vi "Host - Laptop.vi"() -> ()   [LabVIEW 2017]
uses:
  sobot structures/Commands.ctl
  sobot structures/General_Command.ctl
  sobot structures/ReturnDataStatus.ctl
  sobot structures/XY_Commands.ctl
  sobot structures/Z_Command.ctl
  1dab9ac5-030c-4d51-9c07-0e0460f9bdda.vi
  45e61c1e-af3e-4776-95f2-28021f87d7f5.vi
  209d0eb8-92f5-4172-9cd1-3ed4126d6dd2.vi
  fabacc7d-1012-48c4-9930-a2795e4d71c6.vi
  f1c2f41c-6d0d-4fd5-9c33-fd296998c35a.vi
  567dd2d4-847b-4f17-917f-034123e5cef3.vi
  5a9a0e87-71f9-401a-87e2-2bb0dd87a38c.vi
  200908e3-6be4-4c90-a5fc-498c46c2d1bf.vi
  6d8adddc-4429-438c-b8f0-ba7b589ea023.vi
  c3afd2a6-b29d-4eb4-b88f-7abd21b0c47a.vi
  5fae1378-0665-4254-b68d-0e395951aabf.vi
  267ce563-aefe-4b16-b1f3-47eae334334f.vi
  99eac005-18d9-4fd3-997a-104f87d8fe48.vi
  20e12de9-b1e8-45fd-8220-b65a0c4cd02e.vi
  82c37991-5cff-4107-993c-edab275d39a1.vi
  27a68409-aeb0-4d2d-83e9-8f13cebcd619.vi
  de5fd1d6-9d33-402c-82a6-f57f77f69c7e.vi
  29953faf-593d-4707-840b-6a073ddb8916.vi
panel:
  out "Pingtime":i32
  in  "General_Ping":bool
  out "String":string
  in  "ReflectorPosition":i32
  in  "Z_Position":i32
  in  "Z_Focus":bool
  in  "Z_Initialize":bool
  in  "Z_ReflectorPosition":bool
  in  "Z_MoveToPosition":bool
  in  "XY_Unlock Motors":bool
  in  "XY_LockMotors":bool
  in  "XY_MarkTarget":bool
  in  "XY_MoveToPosition":bool
  in  "XY_Initialize":bool
  in  "Coordinate":dbl[](array[numeric])=[0.0, 0.0, 0.0]
  in  "Message":string
  in  "Positon (X / Y)":i32[](array[numeric])
  in  "General_SimpleMessage":bool
  in  "General_Initialize":bool
  in  "General_TransferPoint":bool
  in  "General_StopSobotAutomatic":bool
  in  "General_StartSobotAutomatic":bool
  in  "General_Stop":bool
  # "General"
  # "XY"
  # "Z"
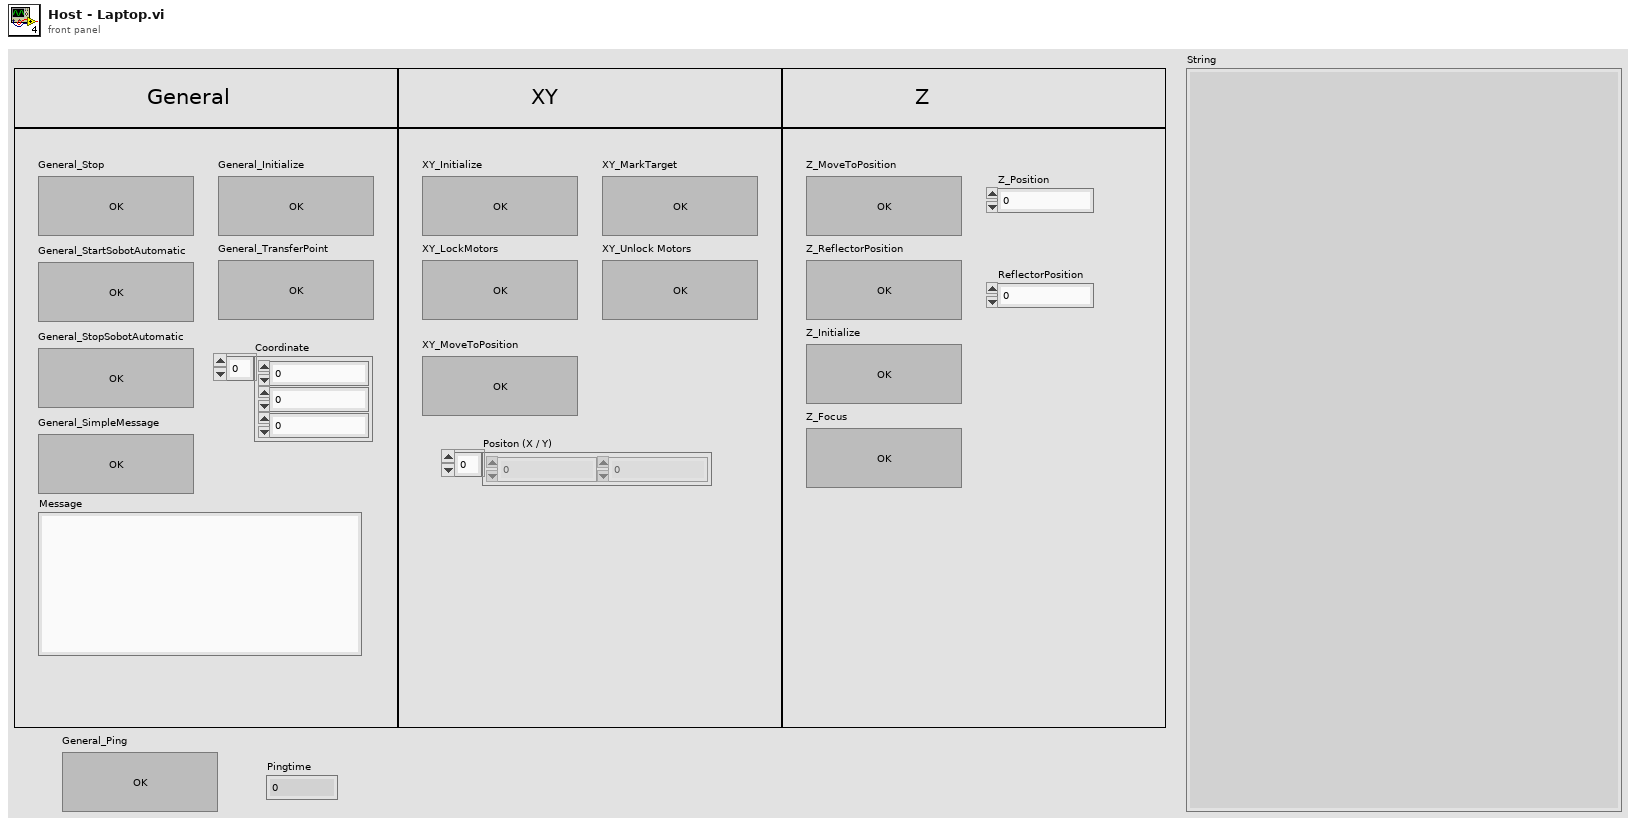
[diagram p1: front panel]
types:
  T1 = typedef "Commands.ctl" = enum16{"General_Stop", "General_StartSobotAutomatic", "General_StopSobotAutomatic", "General_TransferPoint", "General_Initialize", "General_SimpleMessage", "General_Ping", "XY_Initialize", "XY_MoveToPosition", "XY_MarkTarget", "XY_LockMotors", "XY_UnlockMotors", "Z_Initialize", "Z_MoveToPosition", "Z_Focus", "Z_ReflectorPosition", "Plattform_Move", "Plattform_GetDrivingData", "Plattform_GetLivetimeData"}
  T2 = typedef "General_Command.ctl" = enum16{"General_Stop", "General_StartSobotAutomatic", "General_StopSobotAutomatic", "General_TransferPoint", "General_Initialize", "General_SimpleMessage", "General_Ping"}
  T3 = typedef "ReturnDataStatus.ctl" = enum16{"AllOk", "Error"}
  T4 = typedef "XY_Commands.ctl" = enum16{"XY_Initialize", "XY_MoveToPosition", "XY_MarkTarget", "XY_LockMotors", "XY_UnlockMotors"}
  T5 = typedef "Z_Command.ctl" = enum16{"Z_Initialize", "Z_MoveToPosition", "Z_Focus", "Z_ReflectorPosition"}
  T6 = typedef "SoBot_CommandTypes.ctl" = enum16{"General_Command", "XY_Command", "Z_Command", "Plattform_Command"}
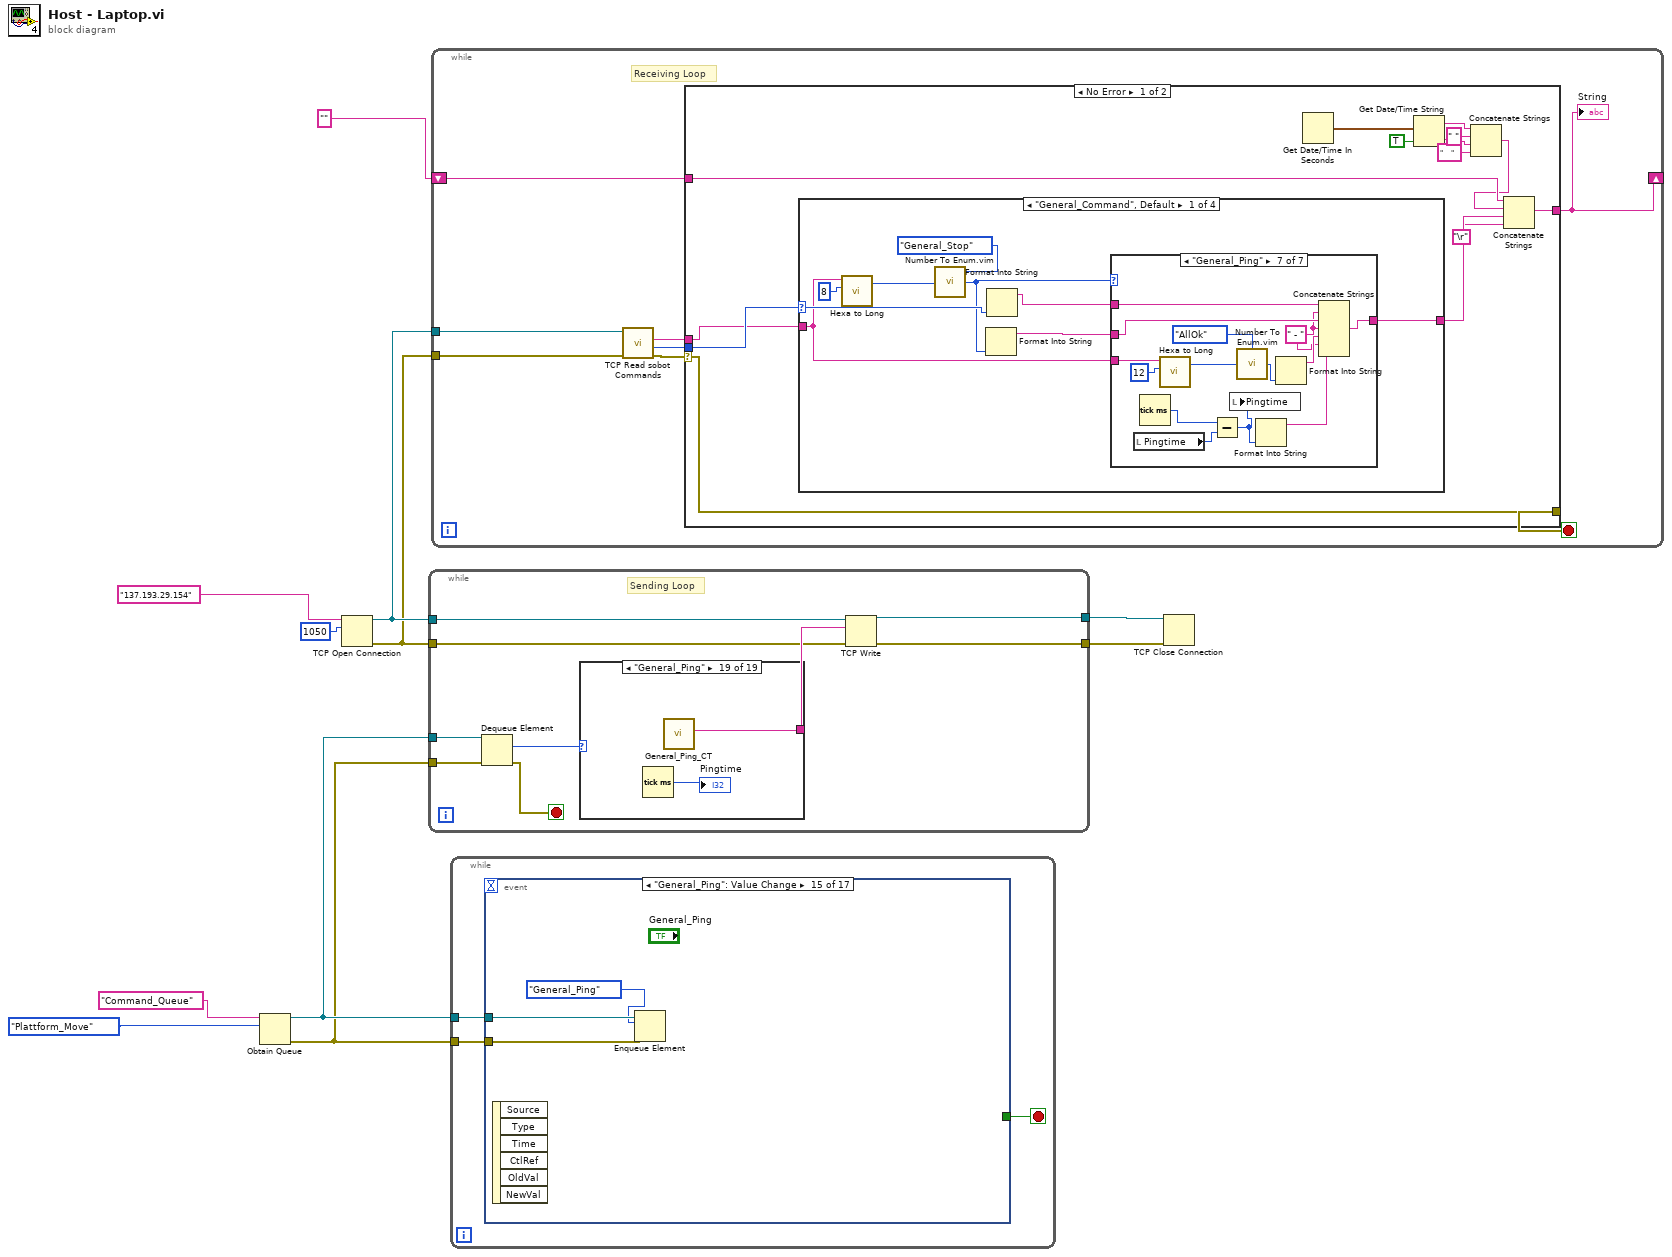
[diagram p0: block diagram]
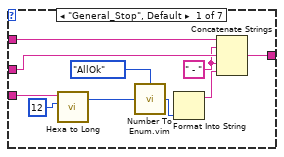
[diagram p2: hidden frame]
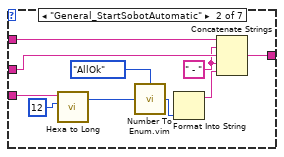
[diagram p3: hidden frame]
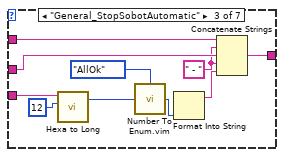
[diagram p4: hidden frame]
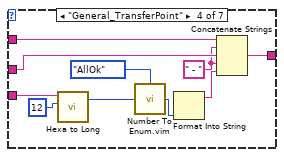
[diagram p5: hidden frame]
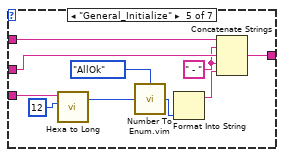
[diagram p6: hidden frame]
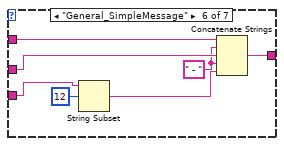
[diagram p7: hidden frame]
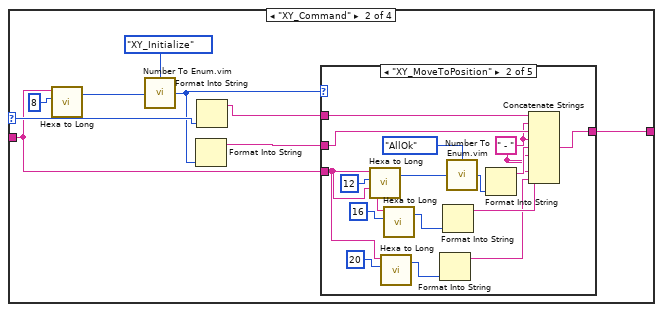
[diagram p8: hidden frame]
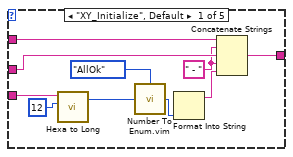
[diagram p9: hidden frame]
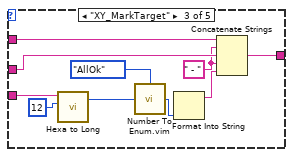
[diagram p10: hidden frame]
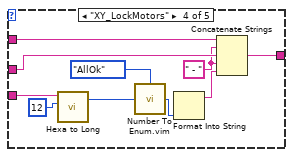
[diagram p11: hidden frame]
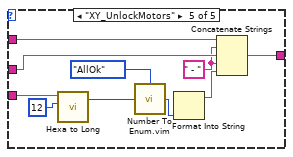
[diagram p12: hidden frame]
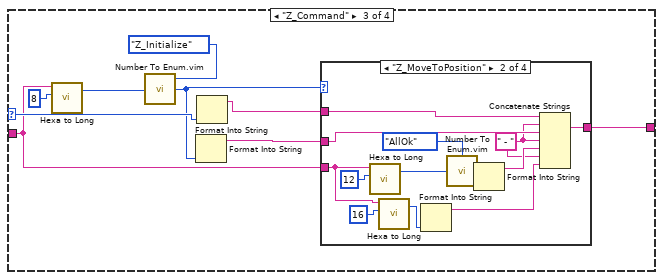
[diagram p13: hidden frame]
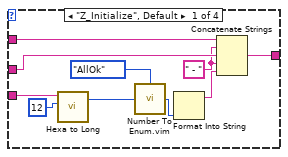
[diagram p14: hidden frame]
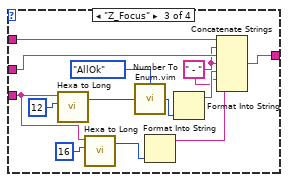
[diagram p15: hidden frame]
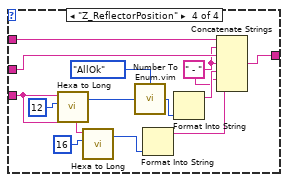
[diagram p16: hidden frame]
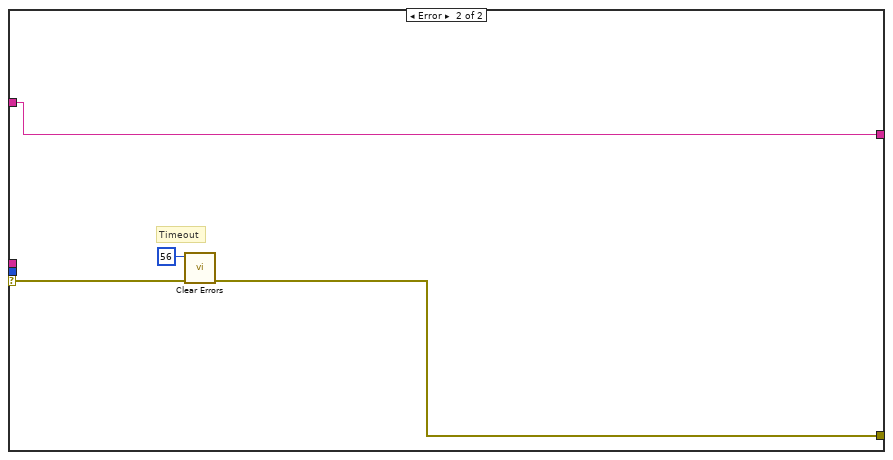
[diagram p18: hidden frame]
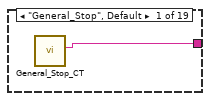
[diagram p19: hidden frame]
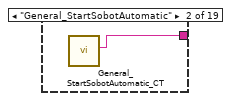
[diagram p20: hidden frame]
diagram:
  n1 = Obtain Queue(name (unnamed)="Command_Queue", element data type=Commands."Plattform_Move") -> (queue out=w7:refnum<queue>, error out=w6:errorcluster)  [unwired: 3 in, 1 out]
  n2 = TCP Open Connection(address="137.193.29.154", remote port or service name=u16 1050) -> (connection ID=w3:refnum<k5>, error out=w2:errorcluster)  [unwired: 3 in]
  n3 = while {
    tunnel: w3 -> [w15]
    tunnel: w2 -> [w14]
    tunnel: w7 -> [w19]
    tunnel: w6 -> [w20]
    tunnel: [w13] -> w5
    tunnel: [w12] -> w4
    stop <- w17 stop-if-true
    # "Sending Loop"
    n4 = Dequeue Element(queue=w19, error in (no error)=w20) -> (element=w18:T1, error out=w17:errorcluster)  [unwired: 1 in, 2 out]
    n5 = case shown="\"General_Ping\"" w18 {
      tunnel: [w21 w22 w23 w25 w26 w28 w29 w31 w32 w33 w34 w35 w37 w38 w40 w41 w42 w43 w45] -> w16
      frame "General_Stop", Default {
        n6 = call "General_Stop_CT.vi"() -> ("Command"=w21:string)  [unwired: 11 in]
      }
      frame "General_StartSobotAutomatic" {
        n7 = call "General_StartSobotAutomatic_CT.vi"() -> ("Command"=w22:string)  [unwired: 11 in]
      }
      frame "General_StopSobotAutomatic" {
        n8 = call "General_StopSobotAutomatic_CT.vi"() -> ("Command"=w23:string)  [unwired: 11 in]
      }
      frame "General_TransferPoint" {
        n9 = call "General_TransferPoint_CT.vi"("Coordinate"="Coordinate") -> ("Command"=w25:string)  [unwired: 10 in]
      }
      frame "General_Initialize" {
        n10 = call "General_Initialize_CT.vi"() -> ("Command"=w26:string)  [unwired: 11 in]
      }
      frame "General_SimpleMessage" {
        n11 = call "General_SimpleMessage_CT.vi"("Message"="Message") -> ("Command"=w28:string)  [unwired: 10 in]
      }
      frame "XY_Initialize" {
        n12 = call "XY_Initialize_CT.vi"() -> ("Command"=w29:string)  [unwired: 11 in]
      }
      frame "XY_MoveToPosition" {
        n13 = call "XY_MoveToPosition_CT.vi"("Positon (X / Y)"="Positon (X / Y)") -> ("Command"=w31:string)  [unwired: 10 in]
      }
      frame "XY_MarkTarget" {
        n14 = call "XY_MarkTarget_CT.vi"() -> ("Command"=w32:string)  [unwired: 11 in]
      }
      frame "XY_LockMotors" {
        n15 = call "XY_LockMotors_CT.vi"() -> ("Command"=w33:string)  [unwired: 11 in]
      }
      frame "XY_UnlockMotors" {
        n16 = call "XY_UnlockMotors_CT.vi"() -> ("Command"=w34:string)  [unwired: 11 in]
      }
      frame "Z_Initialize" {
        n17 = call "Z_Initialize_CT.vi"() -> ("Command"=w35:string)  [unwired: 11 in]
      }
      frame "Z_MoveToPosition" {
        n18 = call "Z_MoveToPosition_CT.vi"("Z_Position"="Z_Position") -> ("Command"=w37:string)  [unwired: 10 in]
      }
      frame "Z_Focus" {
        n19 = call "Z_Focus_CT.vi"() -> ("Command"=w38:string)  [unwired: 11 in]
      }
      frame "Z_ReflectorPosition" {
        n20 = call "Z_ReflectorPosition_CT.vi"("ReflectorPosition"="ReflectorPosition") -> ("Command"=w40:string)  [unwired: 10 in]
      }
      frame "Plattform_Move" {
        n21 = call "Plattform_Move_CT.vi"() -> ("Command"=w41:string)  [unwired: 11 in]
      }
      frame "Plattform_GetDrivingData" {
        n22 = call "Plattform_GetDrivingData_CT.vi"() -> ("Command"=w42:string)  [unwired: 11 in]
      }
      frame "Plattform_GetLivetimeData" {
        n23 = call "Plattform_GetLivetimeData_CT.vi"() -> ("Command"=w43:string)  [unwired: 11 in]
      }
      frame "General_Ping" {
        n24 = Tick Count (ms)() -> (millisecond timer value=→"Pingtime":u32)
        n25 = call "General_Ping_CT.vi"() -> ("Command"=w45:string)  [unwired: 11 in]
      }
    }
    n26 = TCP Write(connection ID=w15, data in=w16, error in (no error)=w14) -> (connection ID out=w12:refnum<k5>, error out=w13:errorcluster)  [unwired: 1 in, 1 out]
  }
  n27 = while {
    tunnel: w3 -> [w53]
    tunnel: w2 -> [w52]
    shift-right: [w47] -> _
    shift-left: "" -> [w46]
    stop <- w49 stop-if-true
    # "Receiving Loop"
    n28 = call "TCP Read sobot Commands.vi"("error in (no error)"=w52, "TCP Network Connection in"=w53) -> ("error out"=w51:errorcluster, "SoBot_CommandTypes"=w48:T6, "data out"=w50:string)  [unwired: 6 in, 1 out]
    n29 = case shown="No Error" w51 {
      selector: w51 -> [w67 w273]
      tunnel: w50 -> [w65 _]
      tunnel: [w67 w272] -> w49
      tunnel: w48 -> [w66 _]
      tunnel: [w64 w271] -> w47
      tunnel: w46 -> [w55 w271]
      frame No Error {
        n30 = case shown="\"General_Command\", Default" w66 {
          selector: w66 -> [w76 w156 w221 _]
          tunnel: w65 -> [w72 w151 w217 _]
          tunnel: [w69 w148 w214 _] -> w63
          frame "General_Command", Default {
            n31 = call "Hexa to Long.vi"("Hexa"=w72, "Index"=8) -> ("Long"=w74:u32)  [unwired: 4 in]
            n32 = call "Number To Enum.vim"("number"=w74, "enum type"=General_Command."General_Stop" ("General_Command")) -> ("number as enum"=w73:T2)
            n33 = Format Into String(w73) -> (resulting string=w70:string)  [unwired: 3 in, 1 out]
            n34 = Format Into String(w76) -> (resulting string=w71:string)  [unwired: 3 in, 1 out]
            n35 = case shown="\"General_Ping\"" w73 {
              tunnel: w72 -> [w85 w95 w105 w115 w125 w128 w146]
              tunnel: w71 -> [w81 w91 w101 w111 w121 w133 w142]
              tunnel: w70 -> [w80 w90 w100 w110 w120 w132 w141]
              tunnel: [w77 w87 w97 w107 w117 w130 w139] -> w69
              frame "General_Stop", Default {
                w79 = " - " ("string")
                n36 = call "Hexa to Long.vi"("Hexa"=w85, "Index"=12) -> ("Long"=w83:u32)  [unwired: 4 in]
                n37 = call "Number To Enum.vim"("number"=w83, "enum type"=ReturnDataStatus."AllOk" ("ReturnDataStatus")) -> ("number as enum"=w82:T3)
                n38 = Format Into String(w82) -> (resulting string=w78:string)  [unwired: 3 in, 1 out]
                n39 = Concatenate Strings(w81, w79, w80, w79, w78) -> (w77:string)
              }
              frame "General_StartSobotAutomatic" {
                w89 = " - " ("string")
                n40 = call "Hexa to Long.vi"("Hexa"=w95, "Index"=12) -> ("Long"=w93:u32)  [unwired: 4 in]
                n41 = call "Number To Enum.vim"("number"=w93, "enum type"=ReturnDataStatus."AllOk" ("ReturnDataStatus")) -> ("number as enum"=w92:T3)
                n42 = Format Into String(w92) -> (resulting string=w88:string)  [unwired: 3 in, 1 out]
                n43 = Concatenate Strings(w91, w89, w90, w89, w88) -> (w87:string)
              }
              frame "General_StopSobotAutomatic" {
                w99 = " - " ("string")
                n44 = call "Hexa to Long.vi"("Hexa"=w105, "Index"=12) -> ("Long"=w103:u32)  [unwired: 4 in]
                n45 = call "Number To Enum.vim"("number"=w103, "enum type"=ReturnDataStatus."AllOk" ("ReturnDataStatus")) -> ("number as enum"=w102:T3)
                n46 = Format Into String(w102) -> (resulting string=w98:string)  [unwired: 3 in, 1 out]
                n47 = Concatenate Strings(w101, w99, w100, w99, w98) -> (w97:string)
              }
              frame "General_TransferPoint" {
                w109 = " - " ("string")
                n48 = call "Hexa to Long.vi"("Hexa"=w115, "Index"=12) -> ("Long"=w113:u32)  [unwired: 4 in]
                n49 = call "Number To Enum.vim"("number"=w113, "enum type"=ReturnDataStatus."AllOk" ("ReturnDataStatus")) -> ("number as enum"=w112:T3)
                n50 = Format Into String(w112) -> (resulting string=w108:string)  [unwired: 3 in, 1 out]
                n51 = Concatenate Strings(w111, w109, w110, w109, w108) -> (w107:string)
              }
              frame "General_Initialize" {
                w119 = " - " ("string")
                n52 = call "Hexa to Long.vi"("Hexa"=w125, "Index"=12) -> ("Long"=w123:u32)  [unwired: 4 in]
                n53 = call "Number To Enum.vim"("number"=w123, "enum type"=ReturnDataStatus."AllOk" ("ReturnDataStatus")) -> ("number as enum"=w122:T3)
                n54 = Format Into String(w122) -> (resulting string=w118:string)  [unwired: 3 in, 1 out]
                n55 = Concatenate Strings(w121, w119, w120, w119, w118) -> (w117:string)
              }
              frame "General_SimpleMessage" {
                w131 = " - " ("string")
                n56 = String Subset(string=w128, offset (0)=12) -> (substring=w127:string)  [unwired: 1 in]
                n57 = Concatenate Strings(w133, w131, w132, w131, w127) -> (w130:string)
              }
              frame "General_Ping" {
                w136 = " - " ("string")
                n58 = local read "Pingtime"() -> (w137:i32)
                n59 = Tick Count (ms)() -> (millisecond timer value=w138:u32)
                n60 = call "Hexa to Long.vi"("Hexa"=w146, "Index"=12) -> ("Long"=w144:u32)  [unwired: 4 in]
                n61 = Subtract(x=w138, y=w137) -> (x-y=w134:u32)
                n62 = local write "Pingtime"(w134) -> ()
                n63 = call "Number To Enum.vim"("number"=w144, "enum type"=ReturnDataStatus."AllOk" ("ReturnDataStatus")) -> ("number as enum"=w143:T3)
                n64 = Format Into String(w134) -> (resulting string=w135:string)  [unwired: 3 in, 1 out]
                n65 = Format Into String(w143) -> (resulting string=w140:string)  [unwired: 3 in, 1 out]
                n66 = Concatenate Strings(w142, w136, w141, w136, w140, w136, w135) -> (w139:string)
              }
            }
          }
          frame "XY_Command" {
            n67 = call "Hexa to Long.vi"("Hexa"=w151, "Index"=8) -> ("Long"=w154:u32)  [unwired: 4 in]
            n68 = call "Number To Enum.vim"("number"=w154, "enum type"=XY_Commands."XY_Initialize" ("XY_Command")) -> ("number as enum"=w152:T4)
            n69 = Format Into String(w152) -> (resulting string=w149:string)  [unwired: 3 in, 1 out]
            n70 = Format Into String(w156) -> (resulting string=w150:string)  [unwired: 3 in, 1 out]
            n71 = case shown="\"XY_MoveToPosition\"" w152 {
              tunnel: w151 -> [w165 w167 w191 w201 w211]
              tunnel: w150 -> [w161 w178 w187 w197 w207]
              tunnel: w149 -> [w160 w177 w186 w196 w206]
              tunnel: [w157 w175 w183 w193 w203] -> w148
              frame "XY_Initialize", Default {
                w159 = " - " ("string")
                n72 = call "Hexa to Long.vi"("Hexa"=w165, "Index"=12) -> ("Long"=w163:u32)  [unwired: 4 in]
                n73 = call "Number To Enum.vim"("number"=w163, "enum type"=ReturnDataStatus."AllOk" ("ReturnDataStatus")) -> ("number as enum"=w162:T3)
                n74 = Format Into String(w162) -> (resulting string=w158:string)  [unwired: 3 in, 1 out]
                n75 = Concatenate Strings(w161, w159, w160, w159, w158) -> (w157:string)
              }
              frame "XY_MoveToPosition" {
                w169 = " - " ("string")
                n76 = call "Hexa to Long.vi"("Hexa"=w167, "Index"=12) -> ("Long"=w180:u32)  [unwired: 4 in]
                n77 = call "Hexa to Long.vi"("Hexa"=w167, "Index"=20) -> ("Long"=w172:u32)  [unwired: 4 in]
                n78 = call "Hexa to Long.vi"("Hexa"=w167, "Index"=16) -> ("Long"=w173:u32)  [unwired: 4 in]
                n79 = Format Into String(w172) -> (resulting string=w168:string)  [unwired: 3 in, 1 out]
                n80 = Format Into String(w173) -> (resulting string=w170:string)  [unwired: 3 in, 1 out]
                n81 = call "Number To Enum.vim"("number"=w180, "enum type"=ReturnDataStatus."AllOk" ("ReturnDataStatus")) -> ("number as enum"=w179:T3)
                n82 = Format Into String(w179) -> (resulting string=w176:string)  [unwired: 3 in, 1 out]
                n83 = Concatenate Strings(w178, w169, w177, w169, w176, w169, w170, w169, w168) -> (w175:string)
              }
              frame "XY_MarkTarget" {
                w185 = " - " ("string")
                n84 = call "Hexa to Long.vi"("Hexa"=w191, "Index"=12) -> ("Long"=w189:u32)  [unwired: 4 in]
                n85 = call "Number To Enum.vim"("number"=w189, "enum type"=ReturnDataStatus."AllOk" ("ReturnDataStatus")) -> ("number as enum"=w188:T3)
                n86 = Format Into String(w188) -> (resulting string=w184:string)  [unwired: 3 in, 1 out]
                n87 = Concatenate Strings(w187, w185, w186, w185, w184) -> (w183:string)
              }
              frame "XY_LockMotors" {
                w195 = " - " ("string")
                n88 = call "Hexa to Long.vi"("Hexa"=w201, "Index"=12) -> ("Long"=w199:u32)  [unwired: 4 in]
                n89 = call "Number To Enum.vim"("number"=w199, "enum type"=ReturnDataStatus."AllOk" ("ReturnDataStatus")) -> ("number as enum"=w198:T3)
                n90 = Format Into String(w198) -> (resulting string=w194:string)  [unwired: 3 in, 1 out]
                n91 = Concatenate Strings(w197, w195, w196, w195, w194) -> (w193:string)
              }
              frame "XY_UnlockMotors" {
                w205 = " - " ("string")
                n92 = call "Hexa to Long.vi"("Hexa"=w211, "Index"=12) -> ("Long"=w209:u32)  [unwired: 4 in]
                n93 = call "Number To Enum.vim"("number"=w209, "enum type"=ReturnDataStatus."AllOk" ("ReturnDataStatus")) -> ("number as enum"=w208:T3)
                n94 = Format Into String(w208) -> (resulting string=w204:string)  [unwired: 3 in, 1 out]
                n95 = Concatenate Strings(w207, w205, w206, w205, w204) -> (w203:string)
              }
            }
          }
          frame "Z_Command" {
            n96 = call "Hexa to Long.vi"("Hexa"=w217, "Index"=8) -> ("Long"=w219:u32)  [unwired: 4 in]
            n97 = call "Number To Enum.vim"("number"=w219, "enum type"=Z_Command."Z_Initialize" ("Z_Command")) -> ("number as enum"=w218:T5)
            n98 = Format Into String(w218) -> (resulting string=w215:string)  [unwired: 3 in, 1 out]
            n99 = Format Into String(w221) -> (resulting string=w216:string)  [unwired: 3 in, 1 out]
            n100 = case shown="\"Z_MoveToPosition\"" w218 {
              tunnel: w217 -> [w230 w232 w245 w258]
              tunnel: w216 -> [w226 w240 w253 w266]
              tunnel: w215 -> [w225 w239 w252 w265]
              tunnel: [w222 w237 w250 w263] -> w214
              frame "Z_Initialize", Default {
                w224 = " - " ("string")
                n101 = call "Hexa to Long.vi"("Hexa"=w230, "Index"=12) -> ("Long"=w228:u32)  [unwired: 4 in]
                n102 = call "Number To Enum.vim"("number"=w228, "enum type"=ReturnDataStatus."AllOk" ("ReturnDataStatus")) -> ("number as enum"=w227:T3)
                n103 = Format Into String(w227) -> (resulting string=w223:string)  [unwired: 3 in, 1 out]
                n104 = Concatenate Strings(w226, w224, w225, w224, w223) -> (w222:string)
              }
              frame "Z_MoveToPosition" {
                w236 = " - " ("string")
                n105 = call "Hexa to Long.vi"("Hexa"=w232, "Index"=12) -> ("Long"=w242:u32)  [unwired: 4 in]
                n106 = call "Hexa to Long.vi"("Hexa"=w232, "Index"=16) -> ("Long"=w234:u32)  [unwired: 4 in]
                n107 = Format Into String(w234) -> (resulting string=w233:string)  [unwired: 3 in, 1 out]
                n108 = call "Number To Enum.vim"("number"=w242, "enum type"=ReturnDataStatus."AllOk" ("ReturnDataStatus")) -> ("number as enum"=w241:T3)
                n109 = Format Into String(w241) -> (resulting string=w238:string)  [unwired: 3 in, 1 out]
                n110 = Concatenate Strings(w240, w236, w239, w236, w238, w236, w233) -> (w237:string)
              }
              frame "Z_Focus" {
                w249 = " - " ("string")
                n111 = call "Hexa to Long.vi"("Hexa"=w245, "Index"=12) -> ("Long"=w255:u32)  [unwired: 4 in]
                n112 = call "Hexa to Long.vi"("Hexa"=w245, "Index"=16) -> ("Long"=w247:u32)  [unwired: 4 in]
                n113 = call "Number To Enum.vim"("number"=w255, "enum type"=ReturnDataStatus."AllOk" ("ReturnDataStatus")) -> ("number as enum"=w254:T3)
                n114 = Format Into String(w247) -> (resulting string=w246:string)  [unwired: 3 in, 1 out]
                n115 = Format Into String(w254) -> (resulting string=w251:string)  [unwired: 3 in, 1 out]
                n116 = Concatenate Strings(w253, w249, w252, w249, w251, w249, w246) -> (w250:string)
              }
              frame "Z_ReflectorPosition" {
                w260 = " - " ("string")
                n117 = call "Hexa to Long.vi"("Hexa"=w258, "Index"=12) -> ("Long"=w268:u32)  [unwired: 4 in]
                n118 = call "Hexa to Long.vi"("Hexa"=w258, "Index"=16) -> ("Long"=w261:u32)  [unwired: 4 in]
                n119 = call "Number To Enum.vim"("number"=w268, "enum type"=ReturnDataStatus."AllOk" ("ReturnDataStatus")) -> ("number as enum"=w267:T3)
                n120 = Format Into String(w261) -> (resulting string=w259:string)  [unwired: 3 in, 1 out]
                n121 = Format Into String(w267) -> (resulting string=w264:string)  [unwired: 3 in, 1 out]
                n122 = Concatenate Strings(w266, w260, w265, w260, w264, w260, w259) -> (w263:string)
              }
            }
          }
          frame "Plattform_Command" {
          }
        }
        n123 = Get Date/Time In Seconds() -> (seconds since 1Jan1904=w61:timestamp)
        n124 = Get Date/Time String(seconds (now)=w61, want seconds? (F)=TRUE) -> (date string=w59:string, time string=w58:string)  [unwired: 1 in]
        n125 = Concatenate Strings(w59, " " ("string"), w58, "    " ("string")) -> (w54:string)
        n126 = Concatenate Strings(w55, w54, w63, "\r") -> (w64:string)
      }
      frame Error {
        # "Timeout"
        n127 = call <vilib>:"Clear Errors.vi"("error in (no error)"=w273, "specific error code to clear (0: all)"=56) -> ("error out"=w272:errorcluster)  [unwired: 4 in, 1 out]
      }
    }
    "String" <- w47
  }
  n128 = while {
    tunnel: w7 -> [w276]
    tunnel: w6 -> [w275]
    stop <- w277 stop-if-true
    n129 = event shown="[14] \"General_Ping\": Value Change" {
      selector: _ -> [_ _ _ _ _ _ _ _ _ _ _ _ _ _ _ _ _]
      dyn-events: _ -> [_ _ _ _ _ _ _ _ _ _ _ _ _ _ _ _ _]
      timeout: _ -> [_ _ _ _ _ _ _ _ _ _ _ _ _ _ _ _ _]
      tunnel: [_ _ _ _ _ TRUE _ _ _ _ _ _ _ _ _ _ _] -> w277
      tunnel: w276 -> [_ w279 w282 w285 w288 w292 w299 w302 w305 w308 w311 w314 w317 w320 w324 w326 w329]
      tunnel: w275 -> [_ w278 w281 w284 w287 w291 w298 w301 w304 w307 w310 w313 w318 w321 w323 w325 w328]
      event Timeout {
        n130 = event-data() -> ()  [unwired: 1 in, 3 out]
      }
      event "Z_Focus": Value Change {
        n131 = event-data() -> ()  [unwired: 1 in, 6 out]
        n132 = Enqueue Element(queue=w279, element=Commands."Z_Focus", error in (no error)=w278) -> ()  [unwired: 1 in, 3 out]
      }
      event "Z_Initialize": Value Change {
        n133 = event-data() -> ()  [unwired: 1 in, 6 out]
        n134 = Enqueue Element(queue=w282, element=Commands."Z_Initialize", error in (no error)=w281) -> ()  [unwired: 1 in, 3 out]
      }
      event "Z_MoveToPosition": Value Change {
        n135 = event-data() -> ()  [unwired: 1 in, 6 out]
        n136 = Enqueue Element(queue=w285, element=Commands."Z_MoveToPosition", error in (no error)=w284) -> ()  [unwired: 1 in, 3 out]
      }
      event "Z_ReflectorPosition": Value Change {
        n137 = event-data() -> ()  [unwired: 1 in, 1 out]
        n138 = Enqueue Element(queue=w288, element=Commands."Z_ReflectorPosition", error in (no error)=w287) -> ()  [unwired: 1 in, 3 out]
      }
      event "General_Stop": Value Change {
        n139 = event-data() -> ()  [unwired: 1 in, 1 out]
        n140 = Enqueue Element(queue=w292, element=General_Command."General_Stop", error in (no error)=w291) -> (queue out=w290:refnum<queue>, error out=w296:errorcluster)  [unwired: 1 in, 1 out]
        n141 = call "Wait Ms.vi"("error in (no error)"=w296, "milliseconds to wait"=u32 1000) -> ("error out"=w294:errorcluster)  [unwired: 9 in]
        n142 = Release Queue(queue=w290, error in (no error)=w294) -> ()  [unwired: 1 in, 3 out]
      }
      event "General_Initialize": Value Change {
        n143 = event-data() -> ()  [unwired: 1 in, 6 out]
        n144 = Enqueue Element(queue=w299, element=General_Command."General_Initialize", error in (no error)=w298) -> ()  [unwired: 1 in, 3 out]
      }
      event "General_StartSobotAutomatic": Value Change {
        n145 = event-data() -> ()  [unwired: 1 in, 6 out]
        n146 = Enqueue Element(queue=w302, element=General_Command."General_StartSobotAutomatic", error in (no error)=w301) -> ()  [unwired: 1 in, 3 out]
      }
      event "General_StopSobotAutomatic": Value Change {
        n147 = event-data() -> ()  [unwired: 1 in, 6 out]
        n148 = Enqueue Element(queue=w305, element=General_Command."General_StopSobotAutomatic", error in (no error)=w304) -> ()  [unwired: 1 in, 3 out]
      }
      event "General_TransferPoint": Value Change {
        n149 = event-data() -> ()  [unwired: 1 in, 6 out]
        n150 = Enqueue Element(queue=w308, element=General_Command."General_TransferPoint", error in (no error)=w307) -> ()  [unwired: 1 in, 3 out]
      }
      event "General_SimpleMessage": Value Change {
        n151 = event-data() -> ()  [unwired: 1 in, 6 out]
        n152 = Enqueue Element(queue=w311, element=General_Command."General_SimpleMessage", error in (no error)=w310) -> ()  [unwired: 1 in, 3 out]
      }
      event "XY_Unlock Motors": Value Change {
        n153 = event-data() -> ()  [unwired: 1 in, 6 out]
        n154 = Enqueue Element(queue=w314, element=Commands."XY_UnlockMotors", error in (no error)=w313) -> ()  [unwired: 1 in, 3 out]
      }
      event "XY_Initialize": Value Change {
        n155 = event-data() -> ()  [unwired: 1 in, 6 out]
        n156 = Enqueue Element(queue=w317, element=Commands."XY_Initialize", error in (no error)=w318) -> ()  [unwired: 1 in, 3 out]
      }
      event "XY_MoveToPosition": Value Change {
        n157 = event-data() -> ()  [unwired: 1 in, 6 out]
        n158 = Enqueue Element(queue=w320, element=Commands."XY_MoveToPosition", error in (no error)=w321) -> ()  [unwired: 1 in, 3 out]
      }
      event "General_Ping": Value Change {
        n159 = event-data() -> ()  [unwired: 1 in, 6 out]
        n160 = Enqueue Element(queue=w324, element=Commands."General_Ping", error in (no error)=w323) -> ()  [unwired: 1 in, 3 out]
      }
      event "XY_MarkTarget": Value Change {
        n161 = event-data() -> ()  [unwired: 1 in, 6 out]
        n162 = Enqueue Element(queue=w326, element=Commands."XY_MarkTarget", error in (no error)=w325) -> ()  [unwired: 1 in, 3 out]
      }
      event "XY_LockMotors": Value Change {
        n163 = event-data() -> ()  [unwired: 1 in, 6 out]
        n164 = Enqueue Element(queue=w329, element=Commands."XY_LockMotors", error in (no error)=w328) -> ()  [unwired: 1 in, 3 out]
      }
    }
  }
  n165 = TCP Close Connection(connection ID=w4, error in (no error)=w5) -> ()  [unwired: 1 in, 2 out]
